vi "Read Variable X Ref.vi"(11 "Conditional Dialog in":refnum<class "Conditional Dialog.lvclass">) -> (2 "Variable X Ref":refnum<vi>, 3 "Conditional Dialog out":refnum<class "Conditional Dialog.lvclass">)   [LabVIEW 2017, in "Conditional Dialog.lvclass"]
uses:
  <vilib>/gpm_packages/@cs/Test-executive-builder/Source/Test Executive Builder Dialogs/Edit Conditional Dialog/Conditional Dialog.lvclass
  <vilib>/gpm_packages/@cs/Test-executive-builder/Source/Test Executive Builder Dialogs/Edit Conditional Dialog/Conditional Dialog.lvclass/Conditional Dialog.ctl
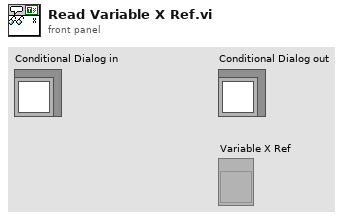
[diagram p1: front panel]
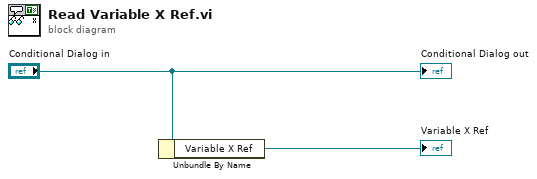
[diagram p0: block diagram]
diagram:
  n1 = Unbundle By Name("Conditional Dialog in") -> ("Variable X Ref"=→"Variable X Ref":refnum<vi>)
  "Conditional Dialog out" <- "Conditional Dialog in"
